vi "SearchingThings.vi"(8 "error in (no error)":errorcluster, 10 "Searching thing":string, 11 "Products":T1[](array[typedef])) -> (0 "error out":errorcluster, 3 "Index of Searching Thing":i32)   [LabVIEW 2022 SP3]
uses:
  #typedef_product.ctl
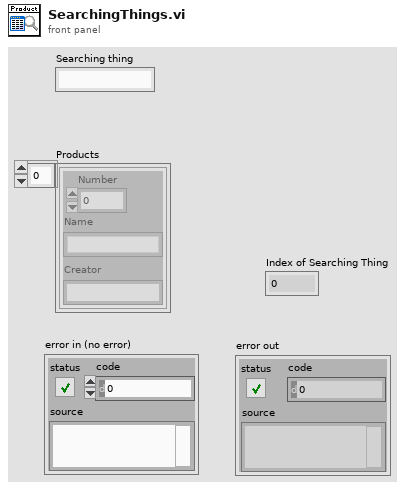
[diagram p1: front panel]
types:
  T1 = typedef "#typedef_product.ctl" = cluster{"Number ":i32, "Name":string, "Creator":string}
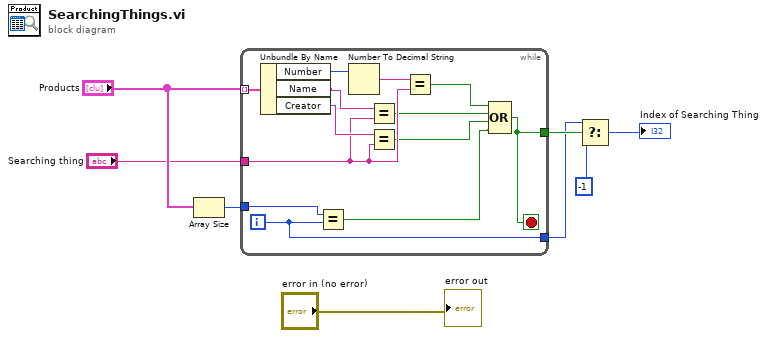
[diagram p0: block diagram]
diagram:
  n1 = Array Size(array="Products") -> (size(s)=w8:i32)
  n2 = while {
    tunnel: "Searching thing" -> [w16]
    tunnel: "Products" -> [w21] mode=indexing
    tunnel: w8 -> [w12]
    tunnel: [w10] -> w2
    tunnel: [w9] -> w3
    i -> [w10]
    stop <- w9 stop-if-true
    n3 = Unbundle By Name(w21) -> ("Number"=w20:i32, "Name"=w18:string, "Creator"=w17:string)
    n4 = Equal?(x=w12, y=w10) -> (x = y?=w11:bool)
    n5 = Number To Decimal String(number=w20) -> (decimal integer string=w19:string)  [unwired: 1 in]
    n6 = Equal?(x=w18, y=w16) -> (x = y?=w14:bool)
    n7 = Equal?(x=w17, y=w16) -> (x = y?=w13:bool)
    n8 = Equal?(x=w19, y=w16) -> (x = y?=w15:bool)
    n9 = Compound Arithmetic op=OR(w15, w14, w13, w11) -> (w9:bool)
  }
  n10 = Select(t=w2, s=w3, f=-1) -> (s? t:f=→"Index of Searching Thing":i32)
  "error out" <- "error in (no error)"
